vi "oa_Data Check [OPS] (N Channels).vi"(0 "resampled signals":cluster{"r0":dbl, "dr":dbl, "Y":dbl[]}[](array[cluster]) {"r0" format="%.2p"; "dr" format="%.2p"; "Y" format="%.2f"}, 1 "restart averaging (F)":bool, 5 "channel info":T1[](array[typedef]) {"channel info"."pregain" format="%.2f"; "channel info"."weighting filter" items=["Linear", "A-weighting", "B-weighting", "C-weighting", "ITU-R 468-4", "Dolby", "CCITT", "C-message", "Wb", "Wc", "Wd", "We", "Wf", "Wh", "Wj", "Wk", "Wm", "AES17 20 kHz lowpass", "AES17 40 kHz lowpass", "AES17 20 kHz highpass", "AES17 40 kHz highpass"]; "channel info"."dB reference" format="%^.1e"; "channel info"."engineering units" items=["custom..."=0, "V"=1, "A"=21, "C"=30, "pC"=31, "s"=32, "-"=29, "Pa"=2, "N"=20, "g"=3, "m/s^2"=4, "m/s"=5, "m"=6, "mm/s"=12, "mm"=13, "micron/s"=14, "micron"=15, "in/s^2"=7, "in/s"=8, "in"=9, "mil/s"=10, "mil"=11, "rad/s^2"=16, "rad/s"=17, "rad"=18, "deg/s^2"=26, "deg/s"=27, "deg"=28, "RPM"=22, "cycle/s^2"=23, "Hz"=24, "cycle"=25, "strain"=19]; "channel info"."sensor sensitivity" format="%#_5f"}, 7 "spectrum settings":cluster{"window type":u32, "block size":i32}={"window type"=1, "block size"=400} {"block size" min=2; "window type" items=["None"=0, "Hanning"=1, "Hamming"=2, "Blackman-Harris"=3, "Exact Blackman"=4, "Blackman"=5, "Flat Top"=6, "4 Term B-Harris"=7, "7 Term B-Harris"=8, "Low Sidelobe"=9, "Gaussian"=62]}, 9 "averaging parameters":T6={"averaging mode"=enum."No averaging", "weighting mode"=enum."Exponential", "number of averages"=10, "linear mode"=enum."One shot"} {"number of averages" min=1 step=1}, 11 "error in (no error)":errorcluster, 12 "processing control in":T5(ring)) -> (4 "dup resampled signals":cluster{"r0":dbl, "dr":dbl, "Y":dbl[]}[](array[cluster]) {"r0" format="%.2p"; "dr" format="%.2p"; "Y" format="%.2f"}, 6 "dup channel info":T1[](array[typedef]) {"channel info"."pregain" format="%.2f"; "channel info"."weighting filter" items=["Linear", "A-weighting", "B-weighting", "C-weighting", "ITU-R 468-4", "Dolby", "CCITT", "C-message", "Wb", "Wc", "Wd", "We", "Wf", "Wh", "Wj", "Wk", "Wm", "AES17 20 kHz lowpass", "AES17 40 kHz lowpass", "AES17 20 kHz highpass", "AES17 40 kHz highpass"]; "channel info"."dB reference" format="%^.1e"; "channel info"."engineering units" items=["custom..."=0, "V"=1, "A"=21, "C"=30, "pC"=31, "s"=32, "-"=29, "Pa"=2, "N"=20, "g"=3, "m/s^2"=4, "m/s"=5, "m"=6, "mm/s"=12, "mm"=13, "micron/s"=14, "micron"=15, "in/s^2"=7, "in/s"=8, "in"=9, "mil/s"=10, "mil"=11, "rad/s^2"=16, "rad/s"=17, "rad"=18, "deg/s^2"=26, "deg/s"=27, "deg"=28, "RPM"=22, "cycle/s^2"=23, "Hz"=24, "cycle"=25, "strain"=19]; "channel info"."sensor sensitivity" format="%#_5f"}, 8 "dup spectrum settings":cluster{"window type":u32, "block size":i32}={"window type"=1, "block size"=400} {"block size" min=2; "window type" items=["None"=0, "Hanning"=1, "Hamming"=2, "Blackman-Harris"=3, "Exact Blackman"=4, "Blackman"=5, "Flat Top"=6, "4 Term B-Harris"=7, "7 Term B-Harris"=8, "Low Sidelobe"=9, "Gaussian"=62]}, 10 "dup averaging parameters":T6={"averaging mode"=enum."No averaging", "weighting mode"=enum."Exponential", "number of averages"=10, "linear mode"=enum."One shot"} {"number of averages" min=1 step=1}, 14 "processing control out":T5(ring), 15 "error out":errorcluster)   [LabVIEW 2017, in "SoundVib_Resampling.lvlib"]
uses:
  <vilib>/addons/Sound and Vibration/Order Analysis/Resample Order Tracking/SoundVib_Resampling.lvlib
  <vilib>/addons/_NISVFA/_Shared subVIs/Controls/svc_Resampled Channel Info.ctl
  <vilib>/addons/_NISVFA/_Shared subVIs/Controls/svc_Channel Info.ctl
  <vilib>/addons/_NISVFA/_Shared subVIs/Controls/svc_Engineering Units Text Ring.ctl
  <vilib>/addons/_NISVFA/_Shared subVIs/Controls/svc_Weighting Filter Text Ring.ctl
  <vilib>/addons/Sound and Vibration/Order Analysis/Resample Order Tracking/SubVIs/OAT Verify Resampled Signal (Multi Channels).vi
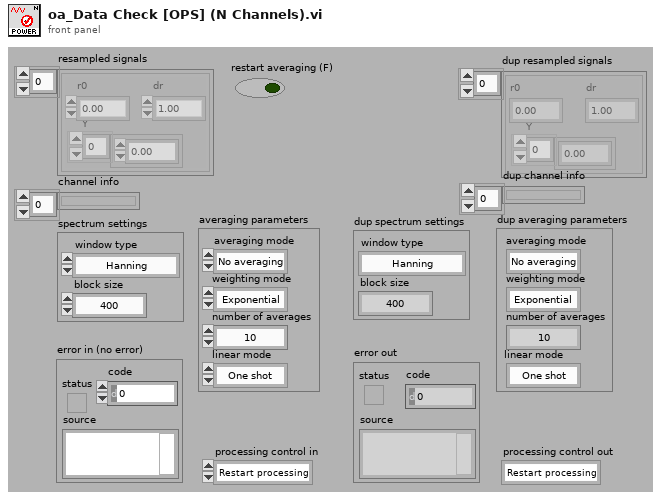
[diagram p1: front panel]
types:
  T1 = typedef "svc_Resampled Channel Info.ctl" = cluster{"channel name":string, "description":string, " channel info":T2}
  T2 = typedef "svc_Channel Info.ctl" = cluster{"sensor sensitivity":dbl, "engineering units":T3, "dB reference":dbl, "custom label":string, "weighting filter":T4, "pregain":dbl}
  T3 = typedef "svc_Engineering Units Text Ring.ctl" = u16
  T4 = typedef "svc_Weighting Filter Text Ring.ctl" = u16
  T5 = enum16{"Restart processing", "Continue processing", "Skip processing"}
  T6 = cluster{"averaging mode":enum16{"No averaging", "Vector averaging", "RMS averaging", "Peak hold"}, "weighting mode":enum16{"Linear", "Exponential"}, "number of averages":u32, "linear mode":enum16{"One shot", "Auto restart"}}
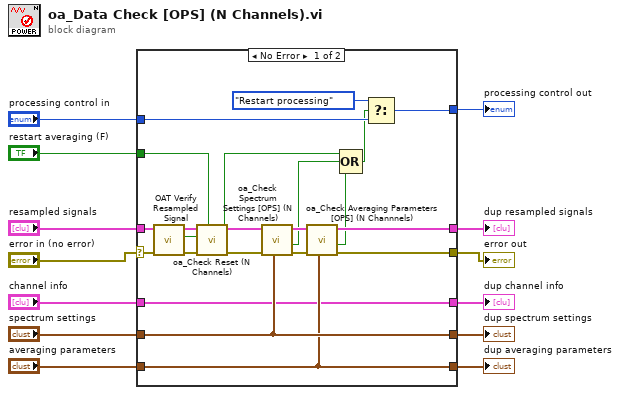
[diagram p0: block diagram]
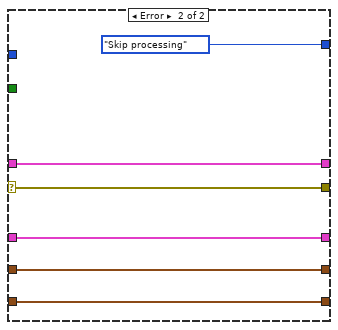
[diagram p2: hidden frame]
diagram:
  n1 = case shown="No Error" "error in (no error)" {
    selector: "error in (no error)" -> [w27 w39]
    tunnel: "resampled signals" -> [w28 w40]
    tunnel: [w29 w40] -> w12
    tunnel: [w35 w39] -> w11
    tunnel: "spectrum settings" -> [w32 w38]
    tunnel: "averaging parameters" -> [w31 w37]
    tunnel: "restart averaging (F)" -> [w17 _]
    tunnel: "processing control in" -> [w34 _]
    tunnel: [w33 T5."Skip processing"] -> w6
    tunnel: [w32 w38] -> w4
    tunnel: [w31 w37] -> w3
    tunnel: "channel info" -> [w30 w36]
    tunnel: [w30 w36] -> w1
    frame No Error {
      n2 = call-poly <vilib>:"OAT Verify Resampled Signal.vi"("error in (no error)"=w27, "resampled signal"=w28) -> ("error out"=w19:errorcluster, "empty signal"=w18:bool, "resampled signal out"=w20:cluster{"r0":dbl, "dr":dbl, "Y":dbl[]}[])  [unwired: 7 in]
      n3 = call <vilib>:"oa_Check Reset (N Channels).vi"("reset?"=w17, "error in (no error)"=w19, "empty?"=w18, "resampled signal"=w20) -> ("error out"=w14:errorcluster, "reset?"=w16:bool, "resampled signal out"=w15:cluster{"r0":dbl, "dr":dbl, "Y":dbl[]}[])  [unwired: 5 in]
      n4 = call <vilib>:"oa_Check Spectrum Settings [OPS] (N Channels).vi"("spectrum settings"=w32, "error in (no error)"=w14, "resampled signals"=w15) -> ("error out"=w25:errorcluster, "parameter changed"=w24:bool, "dup resampled signals"=w26:cluster{"r0":dbl, "dr":dbl, "Y":dbl[]}[])  [unwired: 6 in]
      n5 = call <vilib>:"oa_Check Averaging Parameters [OPS] (N Channnels).vi"("averaging parameters"=w31, "error in (no error)"=w25, "resampled signals"=w26) -> ("error out"=w35:errorcluster, "parameter changed"=w23:bool, "dup resampled signals"=w29:cluster{"r0":dbl, "dr":dbl, "Y":dbl[]}[])  [unwired: 6 in]
      n6 = Compound Arithmetic op=OR(w16, w24, w23) -> (w22:bool)
      n7 = Select(t=T5."Restart processing", s=w22, f=w34) -> (s? t:f=w33:T5)
    }
    frame Error {
    }
  }
  "error out" <- w11
  "dup resampled signals" <- w12
  "dup spectrum settings" <- w4
  "dup averaging parameters" <- w3
  "processing control out" <- w6
  "dup channel info" <- w1
